vi "Rotate Array Benchmark.vi"() -> ()   [LabVIEW 2015]
panel:
  out "Array 2":dbl[](array[numeric])
  out "Times":dbl[](array[numeric])
  in  "Numeric":i32
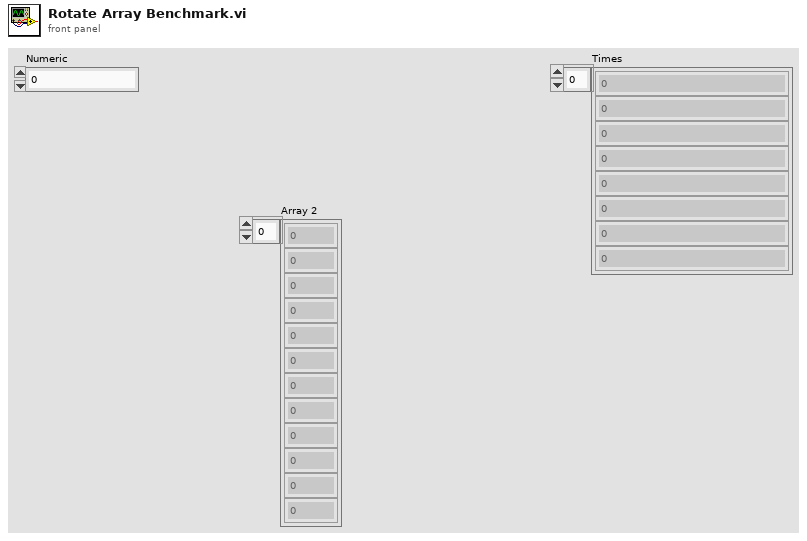
[diagram p1: front panel]
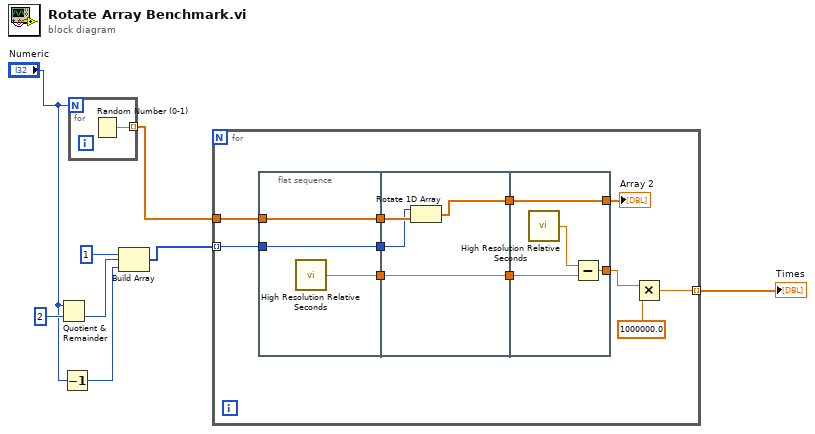
[diagram p0: block diagram]
diagram:
  n1 = Quotient & Remainder(x="Numeric", y=2) -> (floor(x/y)=w6:i32)  [unwired: 1 out]
  n2 = Decrement(x="Numeric") -> (x-1=w4:i32)
  n3 = for {
    N: "Numeric" -> [_]
    tunnel: [w9] -> w2 mode=indexing
    n4 = Random Number (0-1)() -> (number: 0 to 1=w9:dbl)
  }
  n5 = Build Array(1, w6, w4) -> (w3:i32[])
  n6 = for {
    tunnel: w3 -> [w17] mode=indexing
    tunnel: w2 -> [w15]
    tunnel: [w10] -> w1 mode=indexing
    n7 = flat-sequence {
      tunnel: [w23] -> w20
      tunnel: [w22] -> w18
      tunnel: w17 -> [w22]
      tunnel: [w21] -> w16
      tunnel: w15 -> [w21]
      tunnel: w20 -> [w27]
      tunnel: [w27] -> w19
      tunnel: w18 -> [w24]
      tunnel: w16 -> [w26]
      tunnel: [w25] -> w14
      tunnel: w19 -> [w30]
      tunnel: [w29] -> w12
      tunnel: [w28] -> w13
      tunnel: w14 -> [w28]
      frame #0 {
        n8 = call <vilib>:"High Resolution Relative Seconds.vi"() -> ("relative seconds"=w23:dbl)
      }
      frame #1 {
        n9 = Rotate 1D Array(1:w26, 2:w24) -> (0:w25:dbl[])
      }
      frame #2 {
        n10 = call <vilib>:"High Resolution Relative Seconds.vi"() -> ("relative seconds"=w31:dbl)
        n11 = Subtract(x=w31, y=w30) -> (x-y=w29:dbl)
      }
    }
    n12 = Multiply(x=w12, y=1000000.0) -> (x*y=w10:dbl)
    "Array 2" <- w13
  }
  "Times" <- w1
